vi "Cleanup.vi"(8 "error in (no error)":errorcluster, 11 "Coupled Message Rescripter in":refnum<class "Coupled Message Rescripter.lvclass">) -> (0 "error out":errorcluster, 3 "Coupled Message Rescripter out":refnum<class "Coupled Message Rescripter.lvclass">)   [LabVIEW 2020, in "Message Rescripter.lvlib" / "Coupled Message Rescripter.lvclass"]
uses:
  Coupled Message Rescripter.lvclass
  MessageMakerProvider/_Message Maker/_Maker Classes/Coupled Message Scripter/Coupled Message Scripter.lvclass
  Message Rescripter.lvlib
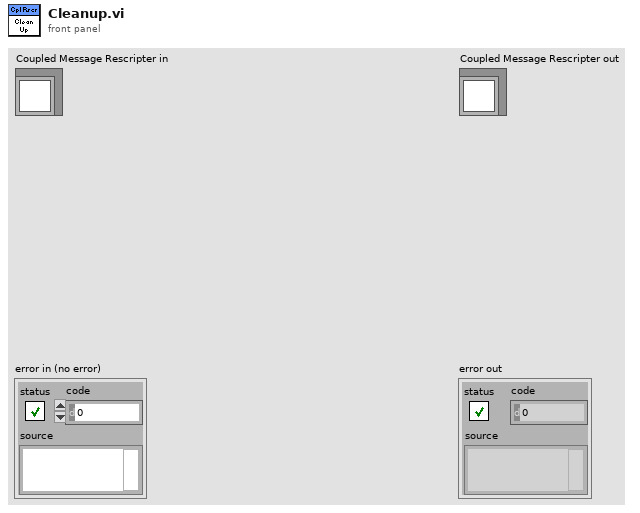
[diagram p1: front panel]
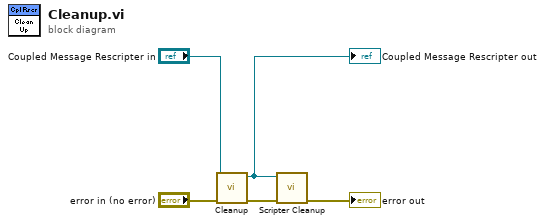
[diagram p0: block diagram]
diagram:
  n1 = call-parent "Cleanup.vi"("error in (no error)"="error in (no error)", "Message Scripter in"="Coupled Message Rescripter in") -> ("error out"=w2:errorcluster, "Message Scripter out"=w3:refnum<class "Coupled Message Rescripter.lvclass">)  [unwired: 8 in]
  "Coupled Message Rescripter out" <- w3
  n2 = call "Scripter Cleanup.vi"("error in (no error)"=w2, "Coupled Message Rescripter in"=w3) -> ("error out"=→"error out":errorcluster)  [unwired: 9 in]
